vi "Read Password file.vi"() -> (4 "Contents":string[][](array[string]))   [LabVIEW 2015]
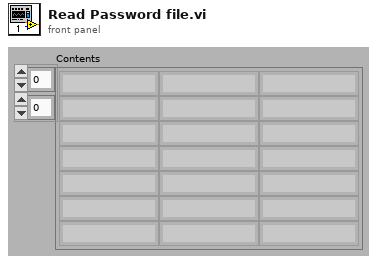
[diagram p1: front panel]
types:
  T1 = enum16{"open", "open or create", "create or replace", "create", "open (read only)"}
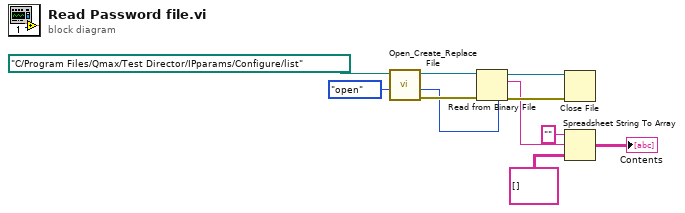
[diagram p0: block diagram]
diagram:
  n1 = call <vilib>:"Open_Create_Replace File.vi"("function (open:0)"=T1."open", "file path"=path "C:/Program Files/Qmax/Test Director/IPparams/Configure/list") -> ("error out"=w11:errorcluster, "file size (bytes)"=w7:i32, "refnum"=w10:refnum<file>)  [unwired: 6 in, 1 out]
  n2 = Read from Binary File(8:w11, 10:w7, 11:w10) -> (0:w9:errorcluster, 2:w6:string, 3:w8:refnum<file>)  [unwired: 3 in, 1 out]
  n3 = Close File(refnum=w8, error in=w9) -> ()  [unwired: 2 out]
  n4 = Spreadsheet String To Array(format string="", spreadsheet string=w6, array type (2D Dbl)=string[][] []) -> (array=→"Contents":string[][])  [unwired: 1 in]
